vi "Check Device.vi"(8 "error in (no error)":errorcluster) -> (0 "error out":errorcluster)   [LabVIEW 2019]
uses:
  cmd_check charge.ctl
  _ctrl/init-r-stop.ctl
  _ctrl/rw.ctl
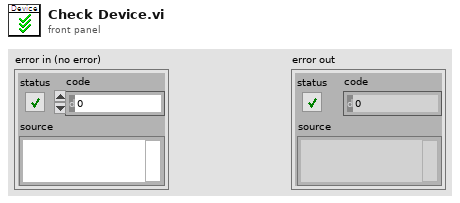
[diagram p1: front panel]
types:
  T1 = typedef "cmd_check charge.ctl" = enum16{"init", "run", "discharge", "disable", "close"}
  T2 = typedef "rw.ctl" = enum16{"read", "write"}
  T3 = typedef "init-r-stop.ctl" = enum16{"ini", "read", "stop"}
  T4 = typedef "Error list.ctl" = cluster{"DL950":bool, "BP4610":bool, "DSP":bool, "AI":bool, "AO":bool, "DO":bool}
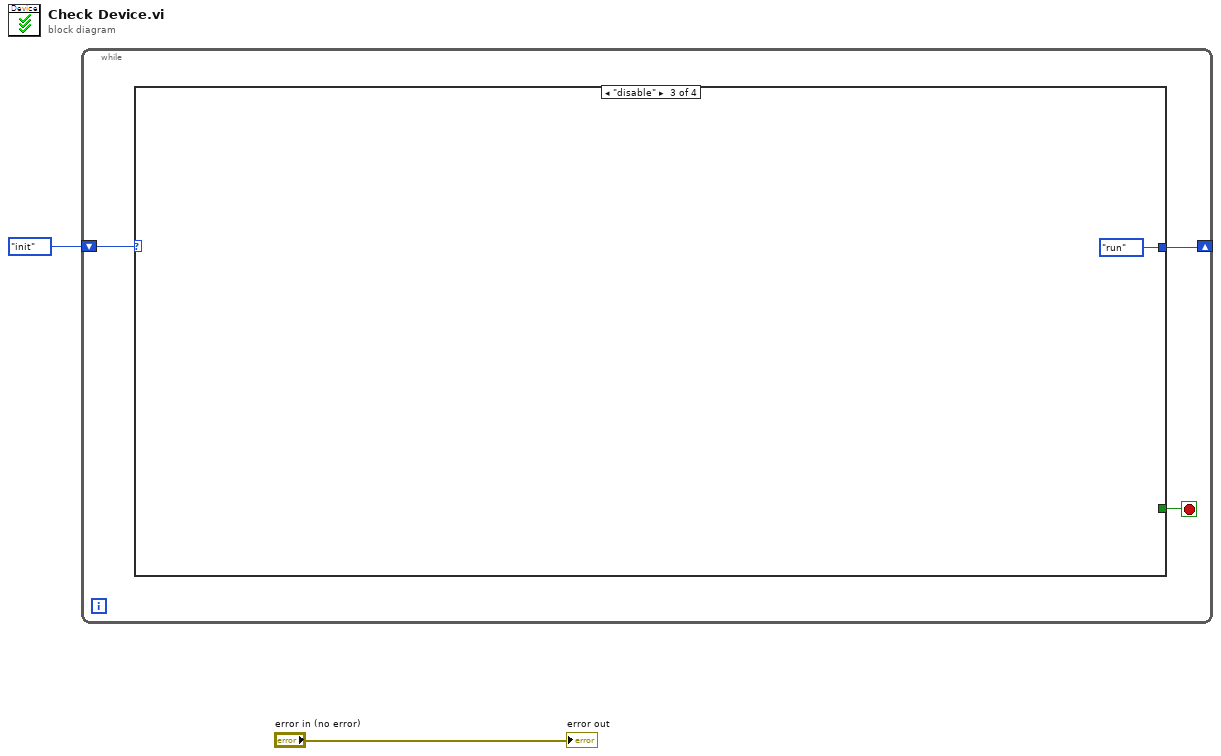
[diagram p0: block diagram]
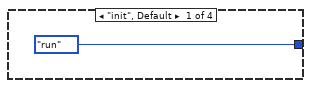
[diagram p2: hidden frame]
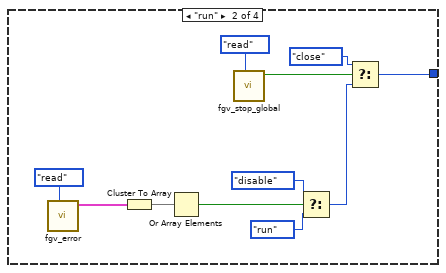
[diagram p3: hidden frame]
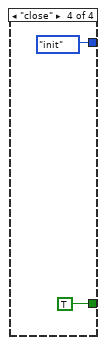
[diagram p4: hidden frame]
diagram:
  n1 = while {
    shift-right: [w4] -> _
    shift-left: cmd_check_charge."init" ("cmd") -> [w5]
    stop <- w3 stop-if-true
    n2 = case shown="\"disable\"" w5 {
      tunnel: [cmd_check_charge."run" ("cmd") w14 cmd_check_charge."run" ("cmd") cmd_check_charge."init" ("cmd")] -> w4
      tunnel: [_ _ _ TRUE] -> w3
      frame "init", Default {
      }
      frame "run" {
        n3 = call "fgv_error.vi"("cmd"=rw."read") -> ("error cluster 2"=w12:T4)  [unwired: 10 in]
        n4 = Cluster To Array(cluster=w12) -> (array=w11:bool[])
        n5 = Or Array Elements(Boolean array=w11) -> (logical OR=w10:bool)
        n6 = call "fgv_stop_global.vi"("cmd"=init-r-stop."read") -> ("stop"=w16:bool)  [unwired: 10 in]
        n7 = Select(t=cmd_check_charge."disable" ("cmd"), s=w10, f=cmd_check_charge."run" ("cmd")) -> (s? t:f=w7:T1)
        n8 = Select(t=cmd_check_charge."close" ("cmd"), s=w16, f=w7) -> (s? t:f=w14:T1)
      }
      frame "disable" {
      }
      frame "close" {
      }
    }
  }
  "error out" <- "error in (no error)"
